vi "AllowContinuousPressureAcquisition.vi"() -> ()   [LabVIEW 2013]
panel:
  in  "AllowContinuousPressureAcqusition":bool
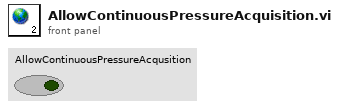
[diagram p1: front panel]
diagram:
